vi "ROIs control menu handler.vi"(9 "ItemTag":string) -> ()   [LabVIEW 2017]
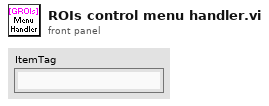
[diagram p1: front panel]
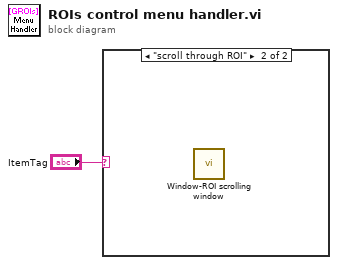
[diagram p0: block diagram]
diagram:
  n1 = case shown="\"scroll through ROI\"" "ItemTag" {
    frame Default {
    }
    frame "scroll through ROI" {
      n2 = call "Window-ROI scrolling window.vi"() -> ()  [unwired: 12 in]
    }
  }
